vi "Fitting-updatecoeff.vi"(0 "Fitting times":i32, 1 "Frame":dbl[](array[numeric]), 2 "X":dbl[](array[numeric]), 3 "Background frame":dbl[](array[numeric]), 4 "Frame error":dbl[](array[numeric]), 5 "Bump":dbl[](array[numeric]), 6 "Upper Limit":dbl[](array[numeric]), 7 "Lower Limit":dbl[](array[numeric]), 8 "Epsilon":dbl, 10 "coeff-a1":dbl, 12 "coeff-a2":dbl, 14 "coeff-a3":dbl, 16 "coeff-a4":dbl) -> (20 "Frame error-output":dbl[](array[numeric]), 21 "Bump-output":dbl[](array[numeric]), 22 "coeff-a1 output":dbl, 23 "coeff-a2 output":dbl, 24 "coeff-a3 output":dbl, 25 "coeff-a4 output":dbl)   [LabVIEW 2015]
uses:
  <vilib>/Analysis/_algsub.llb/Real PseudoInverse Matrix.vi
  <vilib>/Analysis/Matrix/Numeric/Conversions/Array To Matrix - RA.vi
  <vilib>/Analysis/Matrix/Numeric/Conversions/Array To Matrix - RA2.vi
  <vilib>/Analysis/Matrix/Numeric/Multiply/Multiply - RM,RM.vi
  <vilib>/Analysis/Matrix/Numeric/Add/Add - RM,RM.vi
  <vilib>/Analysis/Matrix/Numeric/Conversions/Matrix To Array - RM.vi
  <vilib>/Analysis/NI_AALPro.lvlib
  <vilib>/Analysis/Matrix/NI_Matrix.lvlib
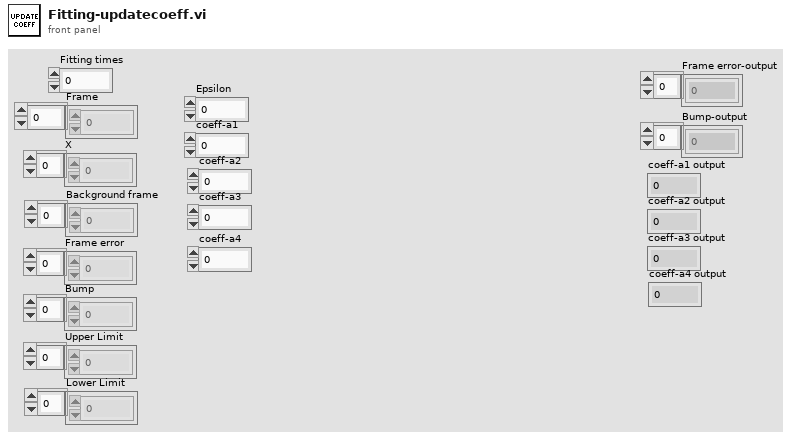
[diagram p1: front panel]
types:
  T1 = typedef "NI_Matrix.lvlib/RealMatrix.ctl" = dbl[][]
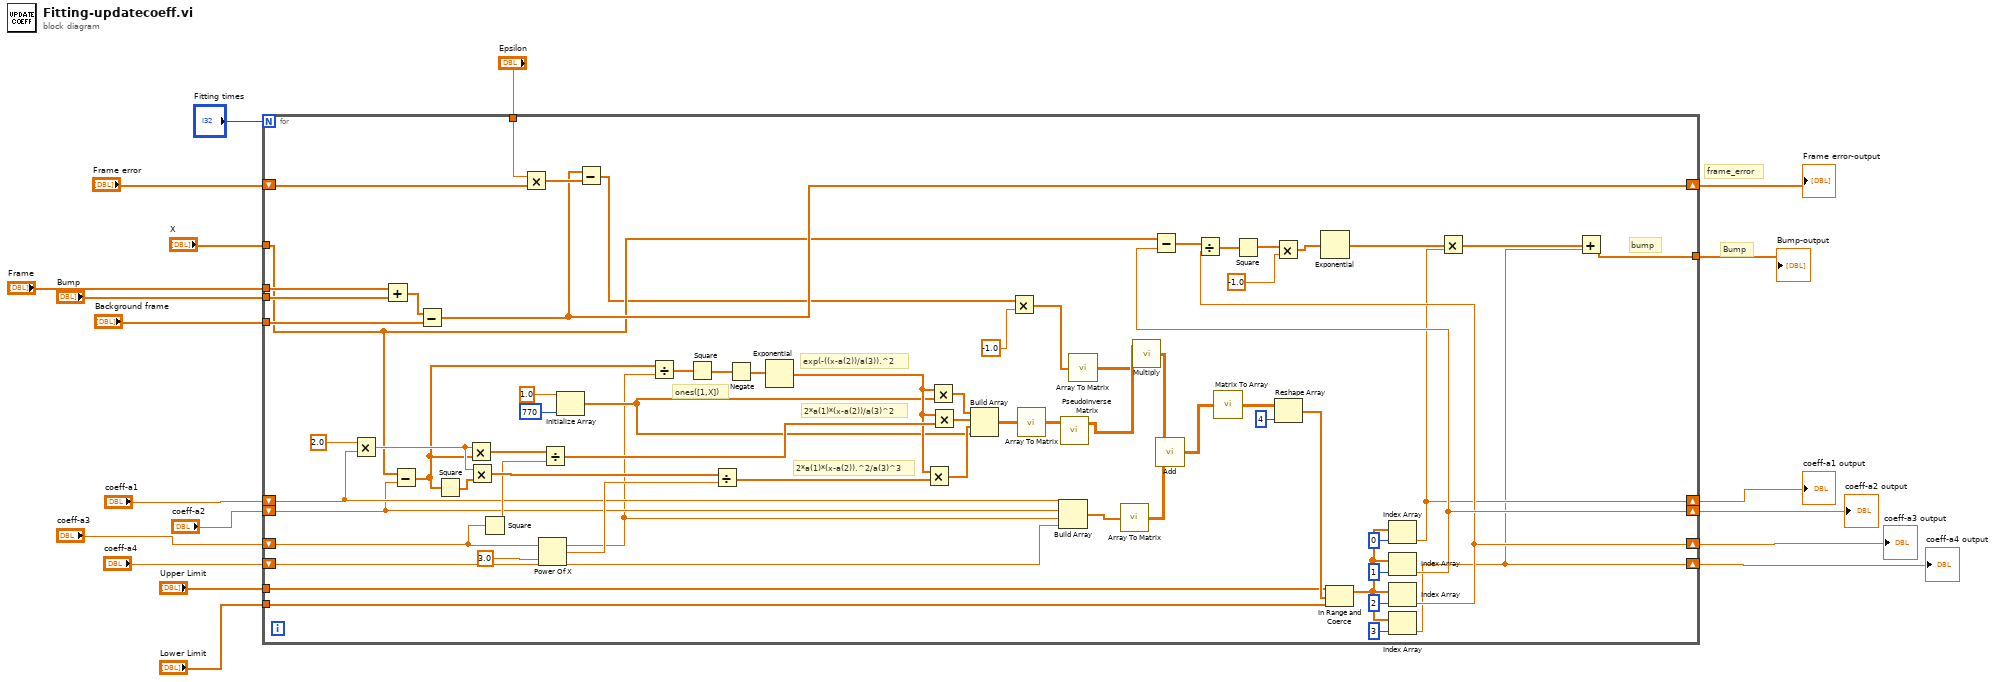
[diagram p0: block diagram]
diagram:
  # "Bump"
  # "frame_error"
  n1 = for {
    N: "Fitting times" -> [_]
    tunnel: "Frame" -> [w86]
    tunnel: "Bump" -> [w85]
    tunnel: "Background frame" -> [w83]
    shift-right: [w79] -> w6
    shift-left: "Frame error" -> [w81]
    tunnel: "Epsilon" -> [w82]
    tunnel: "X" -> [w42]
    shift-right: [w21] -> w4
    shift-left: "coeff-a1" -> [w50]
    shift-right: [w23] -> w3
    shift-left: "coeff-a2" -> [w49]
    shift-right: [w22] -> w2
    shift-left: "coeff-a3" -> [w48]
    shift-right: [w20] -> w1
    shift-left: "coeff-a4" -> [w47]
    tunnel: [w38] -> w5
    tunnel: "Lower Limit" -> [w30]
    tunnel: "Upper Limit" -> [w29]
    # "exp(-((x-a(2))/a(3)).^2"
    # "2*a(1)*(x-a(2))/a(3)^2"
    # "2*a(1)*(x-a(2)).^2/a(3)^3"
    # "bump"
    # "ones([1,X])"
    n2 = Multiply(x=2.0, y=w50) -> (x*y=w74:dbl)
    n3 = Add(x=w86, y=w85) -> (x+y=w84:dbl[])
    n4 = Subtract(x=w42, y=w49) -> (x-y=w69:dbl[])
    n5 = Subtract(x=w84, y=w83) -> (x-y=w79:dbl[])
    n6 = Square(x=w69) -> (x^2=w73:dbl[])
    n7 = Multiply(x=w74, y=w69) -> (x*y=w75:dbl[])
    n8 = Multiply(x=w74, y=w73) -> (x*y=w72:dbl[])
    n9 = Square(x=w48) -> (x^2=w68:dbl)
    n10 = Multiply(x=w82, y=w81) -> (x*y=w80:dbl[])
    n11 = Power Of X(1:3.0 ("x"), 2:w48) -> (0:w70:dbl)
    n12 = Divide(x=w75, y=w68) -> (x/y=w64:dbl[])
    n13 = Initialize Array(1.0 ("element"), 770 ("dimension size")) -> (w58:dbl[])
    n14 = Subtract(x=w79, y=w80) -> (x-y=w35:dbl[])
    n15 = Divide(x=w69, y=w48) -> (x/y=w67:dbl[])
    n16 = Square(x=w67) -> (x^2=w66:dbl[])
    n17 = Divide(x=w72, y=w70) -> (x/y=w62:dbl[])
    n18 = Negate(x=w66) -> (-x=w65:dbl[])
    n19 = Exponential(1:w65) -> (0:w63:dbl[])
    n20 = Multiply(x=w63, y=w62) -> (x*y=w59:dbl[])
    n21 = Multiply(x=w63, y=w58) -> (x*y=w61:dbl[])
    n22 = Multiply(x=w63, y=w64) -> (x*y=w60:dbl[])
    n23 = Build Array(w61, w60, w59, w58) -> (w57:dbl[][])
    n24 = Multiply(x=w35, y=-1.0) -> (x*y=w36:dbl[])
    n25 = call-poly <vilib>:"Array To Matrix.vi"("Real 2D Array"=w57) -> ("Real Matrix"=w56:T1)
    n26 = Build Array(w50, w49, w48, w47) -> (w52:dbl[])
    n27 = call-poly <vilib>:"PseudoInverse Matrix.vi"("Input Matrix"=w56) -> ("PseudoInverse Matrix"=w55:T1)  [unwired: 1 in, 1 out]
    n28 = call-poly <vilib>:"Array To Matrix.vi"("Real 1D Array"=w36) -> ("Real Matrix (Column Vector)"=w54:T1)
    n29 = call-poly <vilib>:"Array To Matrix.vi"("Real 1D Array"=w52) -> ("Real Matrix (Column Vector)"=w51:T1)
    n30 = call-poly <vilib>:"Multiply.vi"("Real Matrix B"=w54, "Real Matrix A"=w55) -> ("A * B"=w53:T1)
    n31 = call-poly <vilib>:"Add.vi"("Real Matrix B"=w51, "Real Matrix A"=w53) -> ("A + B"=w34:T1)
    n32 = call-poly <vilib>:"Matrix To Array.vi"("Real Matrix"=w34) -> ("Real 2D Array"=w33:dbl[][])
    n33 = Reshape Array(w33, 4 ("dimension size")) -> (w31:dbl[])
    n34 = In Range and Coerce(upper limit=w29, x=w31, lower limit=w30) -> (coerced(x)=w28:dbl[])  [unwired: 1 out]
    n35 = Index Array(array=w28, index=0) -> (element=w21:dbl)
    n36 = Index Array(array=w28, index=1) -> (element=w23:dbl)
    n37 = Subtract(x=w42, y=w23) -> (x-y=w46:dbl[])
    n38 = Index Array(array=w28, index=2) -> (element=w22:dbl)
    n39 = Divide(x=w46, y=w22) -> (x/y=w45:dbl[])
    n40 = Square(x=w45) -> (x^2=w44:dbl[])
    n41 = Multiply(x=w44, y=-1.0) -> (x*y=w43:dbl[])
    n42 = Exponential(1:w43) -> (0:w40:dbl[])
    n43 = Index Array(array=w28, index=3) -> (element=w20:dbl)
    n44 = Multiply(x=w40, y=w21) -> (x*y=w39:dbl[])
    n45 = Add(x=w39, y=w20) -> (x+y=w38:dbl[])
  }
  "Frame error-output" <- w6
  "Bump-output" <- w5
  "coeff-a1 output" <- w4
  "coeff-a2 output" <- w3
  "coeff-a3 output" <- w2
  "coeff-a4 output" <- w1
